vi "Caller DVR.vi"(0 "DVR In":refnum<data-value>, 5 "Sub Panel":refnum<vi>, 11 "Error In":errorcluster) -> (4 "DVR Out":refnum<data-value>, 15 "Error Out":errorcluster)   [LabVIEW 2023, in "Arithemetic Operation.lvclass"]
doc: "The method acts as a wrapper to the over riding caller method to call the UI in the sub panel asynchronously."
uses:
  Arithemetic Operation.lvclass
  Typedef/User Event Operations.ctl
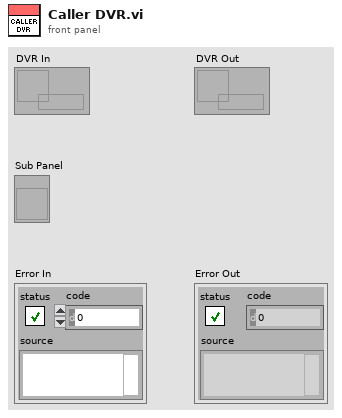
[diagram p1: front panel]
types:
  T1 = typedef "User Event Operations.ctl" = enum16{"Obtain", "Generate", "Release"}
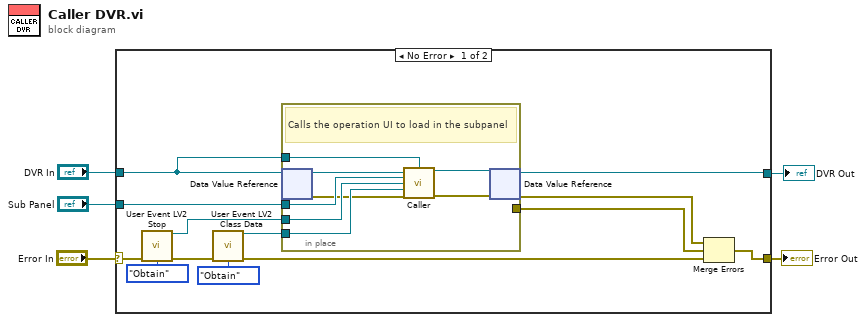
[diagram p0: block diagram]
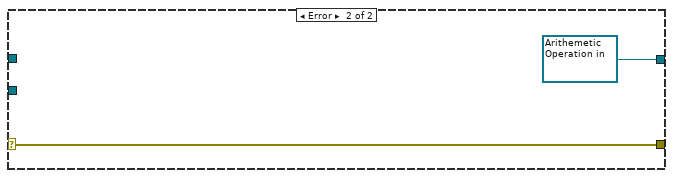
[diagram p2: hidden frame]
diagram:
  n1 = case shown="No Error" "Error In" {
    selector: "Error In" -> [w18 w28]
    tunnel: [w7 w28] -> w4
    tunnel: [w17 refnum<data-value> refnum ("Input")] -> w2
    tunnel: "DVR In" -> [w6 _]
    tunnel: "Sub Panel" -> [w16 _]
    frame No Error {
      n2 = call "User Event LV2 Stop.vi"("Error In"=w18, "Operation"=User_Event_Operations."Obtain") -> ("User Event Ref"=w11:refnum<user-event>, "Error Out"=w13:errorcluster)  [unwired: 12 in]
      n3 = call "User Event LV2 Class Data.vi"("Error In"=w13, "Operation"=User_Event_Operations."Obtain") -> ("User Event Ref"=w15:refnum<user-event>, "Error Out"=w8:errorcluster)  [unwired: 12 in]
      n4 = in-place {
        in-place-border: w16 -> [w24]
        in-place-border: w11 -> [w23]
        in-place-border: w15 -> [w22]
        in-place-border: [w20] -> w9
        in-place-border: w6 -> [w19]
        # "Calls the operation UI to load in the subpanel"
        n5 = in-place-dvr #1(w6) -> (w26:refnum<class "Arithemetic Operation.lvclass">, w21:errorcluster)
        n6 = call-dynamic "Caller.vi"("Arithemetic Operation in"=w26, "DVR"=w19, "Sub Panel"=w24, "State"=w23, "Class Data"=w22, "Error In"=w21) -> ("Arithemetic Operation out"=w25:refnum<class "Arithemetic Operation.lvclass">, "Error Out"=w20:errorcluster)  [unwired: 8 in]
        n7 = in-place-dvr #1(w25) -> (w17:refnum<data-value>, w10:errorcluster)
      }
      n8 = Merge Errors(w10, w9, w8) -> (w7:errorcluster)
    }
    frame Error {
    }
  }
  "Error Out" <- w4
  "DVR Out" <- w2
